vi "File-Settings-Dialog.vi"(8 "error in (no error)":errorcluster) -> (0 "error out":errorcluster, 3 "Process Name Out":string)   [LabVIEW 2018]
panel:
  in  "Notebook Number":string
  in  "Accept":bool
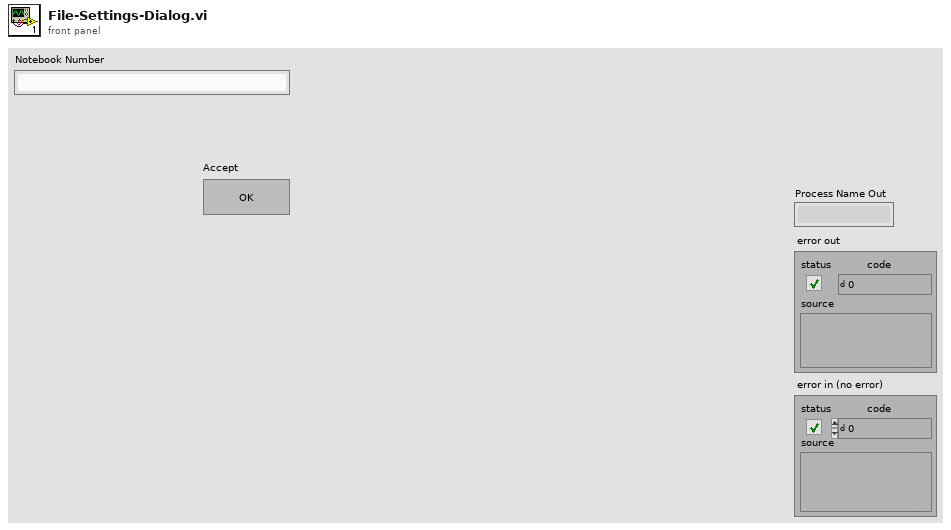
[diagram p1: front panel]
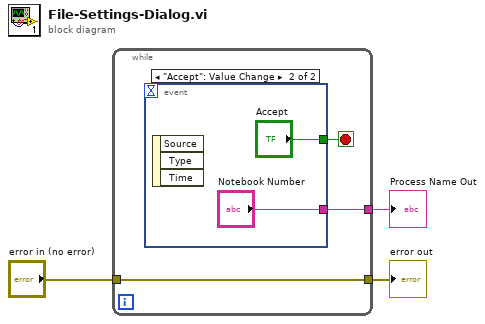
[diagram p0: block diagram]
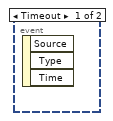
[diagram p2: hidden frame]
diagram:
  n1 = while {
    tunnel: [w6] -> w3
    tunnel: "error in (no error)" -> [w6]
    tunnel: [w4] -> w1
    stop <- w5 stop-if-true
    n2 = event shown="[1] \"Accept\": Value Change" {
      selector: _ -> [_ _]
      dyn-events: _ -> [_ _]
      timeout: _ -> [_ _]
      tunnel: [_ "Notebook Number"] -> w4
      tunnel: [_ "Accept"] -> w5
      event Timeout {
        n3 = event-data() -> ()  [unwired: 1 in, 3 out]
      }
      event "Accept": Value Change {
        n4 = event-data() -> ()  [unwired: 1 in, 3 out]
      }
    }
  }
  "error out" <- w3
  "Process Name Out" <- w1
